vi "Read Active Rectangle.vi"(8 "error in (no error)":errorcluster, 11 "Setting Database in":refnum<class "Setting Database.lvclass">) -> (0 "error out":errorcluster, 2 "Active Rectangle":refnum<class "Rectangle Settings.lvclass">, 3 "Setting Database out":refnum<class "Setting Database.lvclass">)   [LabVIEW 2019, in "Setting Database.lvclass"]
uses:
  Setting Database.lvclass
  Rectangle Settings/Rectangle Settings.lvclass
  Setting Database.lvclass/Setting Database.ctl
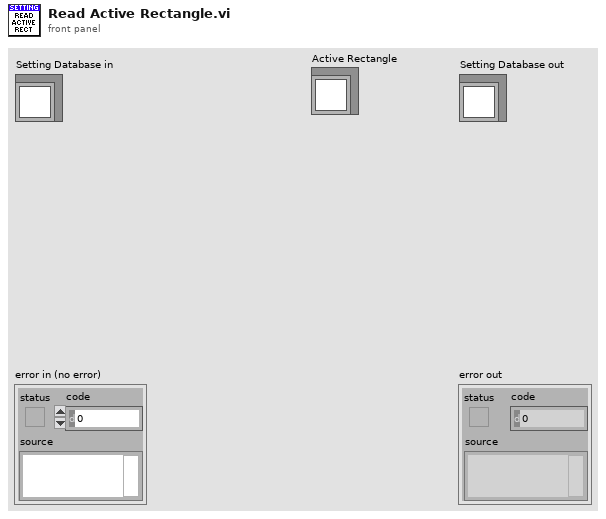
[diagram p1: front panel]
types:
  T1 = cluster{"Path":i32, "Funnel":i32, "Rectangle":i32, "Dot":i32}
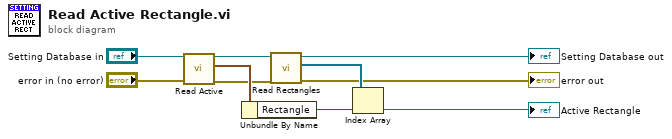
[diagram p0: block diagram]
diagram:
  n1 = call "Read Active.vi"("error in (no error)"="error in (no error)", "Setting Database in"="Setting Database in") -> ("error out"=w2:errorcluster, "Active"=w5:T1, "Setting Database out"=w6:refnum<class "Setting Database.lvclass">)  [unwired: 7 in]
  n2 = Unbundle By Name(w5) -> ("Rectangle"=w4:i32)
  n3 = call "Read Rectangles.vi"("error in (no error)"=w2, "Setting Database in"=w6) -> ("error out"=→"error out":errorcluster, "Rectangles"=w9:refnum<class "Rectangle Settings.lvclass">[], "Setting Database out"=→"Setting Database out":refnum<class "Setting Database.lvclass">)  [unwired: 7 in]
  n4 = Index Array(array=w9, index=w4) -> (element=→"Active Rectangle":refnum<class "Rectangle Settings.lvclass">)
